vi "GV Npix.vi"() -> ()   [LabVIEW 2017]
panel:
  out "Npix max":u16
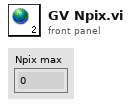
[diagram p1: front panel]
diagram:
